vi "OpenROIImage.vi"(11 "Image  in":T1 {"Dialogs" format="%.0b"}) -> (1 "image":picture, 3 "Image  out":T1 {"Dialogs" format="%.0b"})   [LabVIEW 2019]
uses:
  <userlib>/ImageProcessing/QTLIB_2595_LV86/QT_Image.ctl
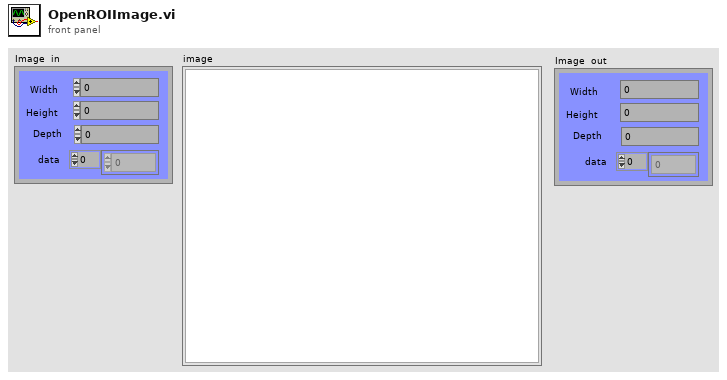
[diagram p1: front panel]
types:
  T1 = typedef "QT_Image.ctl" = cluster{"Width":i32, "Height":i32, "Depth":i32, "data":u8[], "Compressed data":u8[], "Color table":u32[], "Duration":i32, "Options":i32, "Timestamp":i32, "ID":i32, "Reserved":i32, "Dialogs":u32}
  T2 = cluster{"left":i16, "top":i16, "right":i16, "bottom":i16}
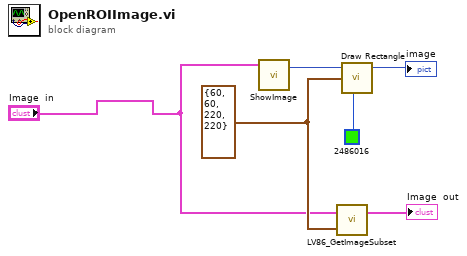
[diagram p0: block diagram]
diagram:
  w3 = T2 {"left"=60, "top"=60, "right"=220, "bottom"=220} ("ROI In")
  n1 = call <userlib>:"ShowImage.vi"("Image"="Image  in") -> ("image"=w4:picture)  [unwired: 2 in, 1 out]
  n2 = call <userlib>:"LV86_GetImageSubset.vi"("ROI"=w3, "Image In"="Image  in") -> ("Image out"=→"Image  out":T1)  [unwired: 1 in]
  n3 = call <vilib>:"Draw Rectangle.vi"("picture"=w4, "rect"=w3, "color(black)"=u32 2486016) -> ("new picture"=→"image":picture)  [unwired: 6 in]
